vi "load modules.vi"() -> ()   [LabVIEW 2012]
uses:
  GFG/GFGstringGet.vi
  GFG/GFG library.lvlib
panel:
  out "Array":T1(array[cluster])
  out "error out":errorcluster
  in  "error in (no error)":errorcluster
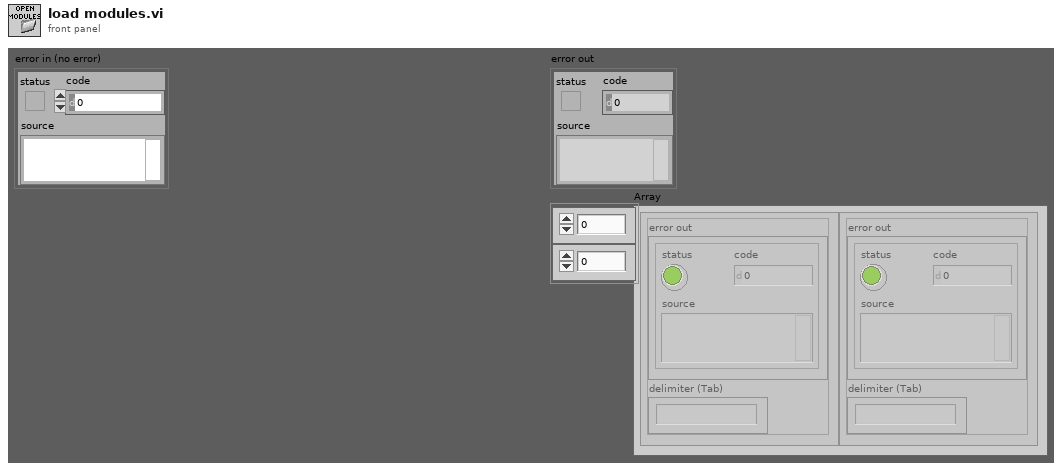
[diagram p1: front panel]
types:
  T1 = cluster{"error out":errorcluster, "delimiter (Tab)":string}[][]
  T2 = enum32{"Invalid", "Standard", "Closed", "Hidden", "Minimized", "Maximized"}
  T3 = cluster{"error out":errorcluster, "delimiter (Tab)":string}
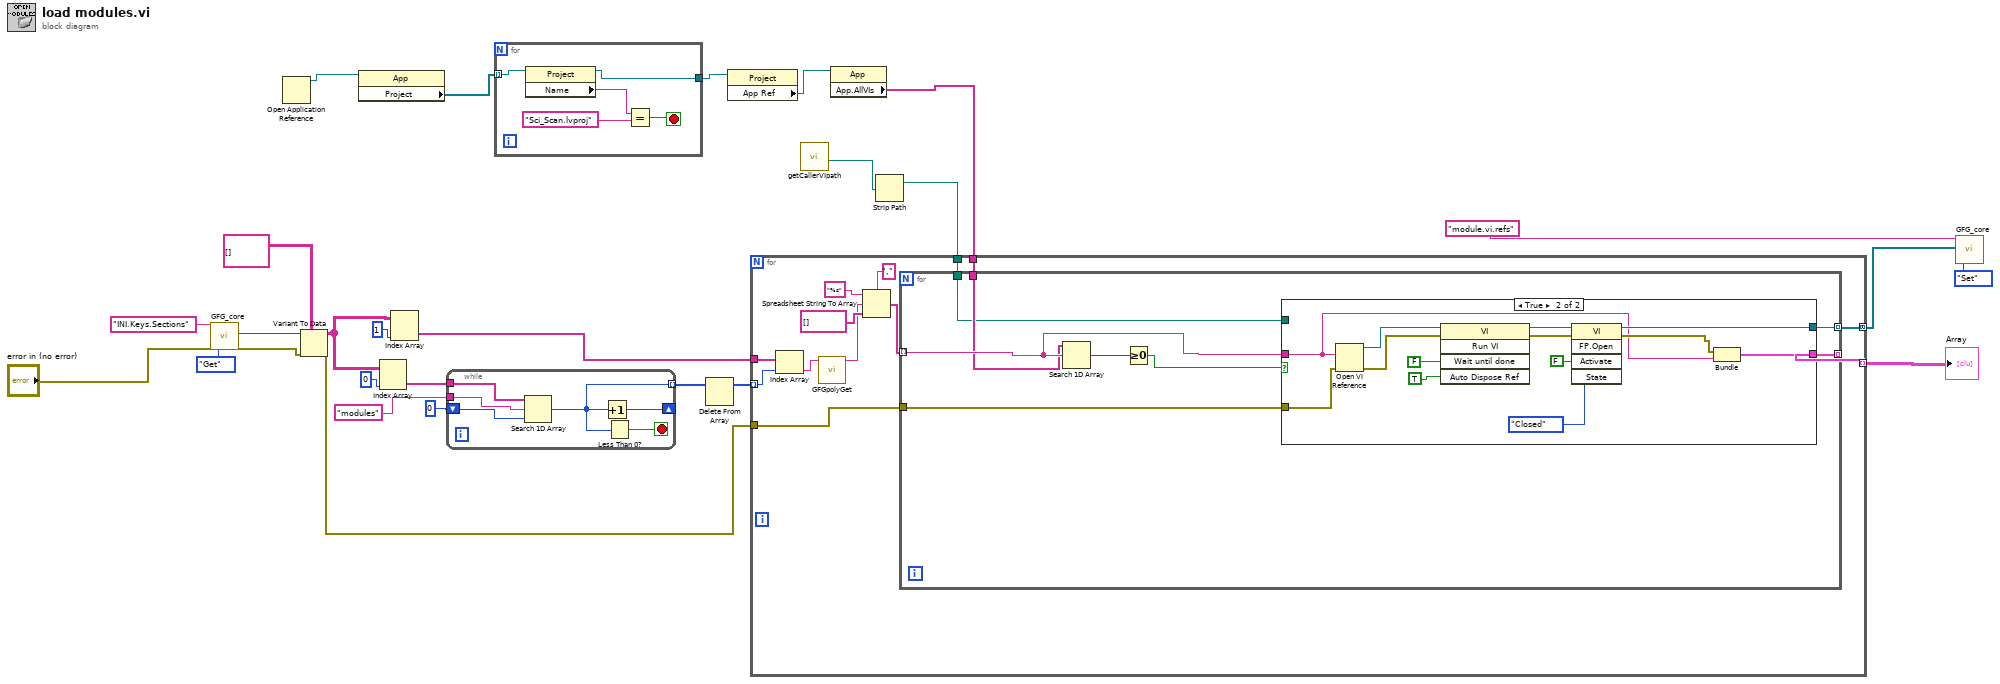
[diagram p0: block diagram]
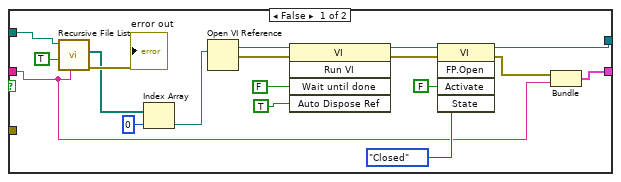
[diagram p2: hidden frame]
diagram:
  n1 = call "GFG_core.vi"("Variable Name in"="INI.Keys.Sections", "error in (no error)"="error in (no error)", "Action"=enum16{"Init", "Set", "Get"}."Get") -> ("Variant Out"=w25:variant, "error out"=w13:errorcluster)  [unwired: 10 in, 5 out]
  n2 = Open Application Reference() -> (3:w2:refnum<vi>)  [unwired: 4 in, 1 out]
  n3 = Variant To Data(error in=w13, type=string[][] [], Variant=w25) -> (data=w21:string[][], error out=w12:errorcluster)
  n4 = property class="App"(reference=w2) -> ("Project"=w3:refnum<vi>[])  [unwired: 1 in, 2 out]
  n5 = Index Array(array=w21, index (col)=0 ("index (row)")) -> (element=w23:string[])  [unwired: 1 in]
  n6 = Index Array(array=w21, index (col)=1 ("index (row)")) -> (element=w20:string[])  [unwired: 1 in]
  n7 = while {
    tunnel: w23 -> [w33]
    shift-right: [w30] -> _
    shift-left: 0 ("index of element") -> [w32]
    tunnel: [w29] -> w16 mode=indexing
    tunnel: "modules" ("element") -> [w28]
    stop <- w31 stop-if-true
    n8 = Search 1D Array(1D array=w33, element=w28, start index (0)=w32) -> (index of element=w29:i32)
    n9 = Increment(x=w29) -> (x+1=w30:i32)
    n10 = Less Than 0?(x=w29) -> (x < 0?=w31:bool)
  }
  n11 = for {
    tunnel: w3 -> [w38] mode=indexing
    tunnel: [w35] -> w4
    stop <- w34 stop-if-true
    n12 = property class="Project"(reference=w38) -> (reference out=w35:refnum<vi>, "Name"=w36:string)  [unwired: 1 in, 1 out]
    n13 = Equal?(x=w36, y="Sci_Scan.lvproj" ("Name")) -> (x = y?=w34:bool)
  }
  n14 = Delete From Array(array=w16) -> (array with subset deleted=w15:i32[])  [unwired: 2 in, 1 out]
  n15 = property class="Project"(reference=w4) -> ("App Ref"=w5:refnum<vi>)  [unwired: 1 in, 2 out]
  n16 = call "getCallerVIpath.vi"() -> ("calling VI's  parent path"=w7:path)  [unwired: 10 in, 1 out]
  n17 = property class="App"(reference=w5) -> ("App.AllVIs"=w1:string[])  [unwired: 1 in, 2 out]
  n18 = Strip Path(path=w7) -> (stripped path=w6:path)  [unwired: 1 out]
  n19 = for {
    tunnel: w20 -> [w51]
    tunnel: w15 -> [w50] mode=indexing
    tunnel: w12 -> [w49]
    tunnel: [w42] -> w10 mode=concatenating
    tunnel: w6 -> [w41]
    tunnel: [w40] -> w8 mode=indexing
    tunnel: w1 -> [w39]
    n20 = Index Array(array=w51, index=w50) -> (element=w44:string)
    n21 = call-poly "GFGpolyGet.vi"("Variable Name in"=w44) -> ("String"=w43:string)  [unwired: 10 in]
    n22 = Spreadsheet String To Array(delimiter (Tab)=",", format string="%s" ("Variable Name in"), spreadsheet string=w43, array type (2D Dbl)=string[] [] ("Array")) -> (array=w45:string[])
    n23 = for {
      tunnel: w49 -> [w54]
      tunnel: w45 -> [w57] mode=indexing
      tunnel: [w59] -> w42 mode=indexing
      tunnel: w41 -> [w53]
      tunnel: [w58] -> w40 mode=indexing
      tunnel: w39 -> [w56]
      n24 = Search 1D Array(1D array=w56, element=w57) -> (index of element=w52:i32)  [unwired: 1 in]
      n25 = Greater Or Equal To 0?(x=w52) -> (x >= 0?=w55:bool)
      n26 = case shown="True" w55 {
        tunnel: w54 -> [_ w86]
        tunnel: [w61 w85] -> w59
        tunnel: [w60 w84] -> w58
        tunnel: w57 -> [w62 w78]
        tunnel: w53 -> [w73 _]
        frame False {
          n27 = call <vilib>:"Recursive File List.vi"("pattern"=w62, "Continue Recursing on Error? (F)"=TRUE, "Folder Path"=w73) -> ("error out"=→"error out":errorcluster, "All Files in Dir"=w75:path[])  [unwired: 4 in, 3 out]
          n28 = Index Array(array=w75, index=0) -> (element=w63:path)
          n29 = Open VI Reference(vi path=w63) -> (vi reference=w67:refnum<vi>, error out=w72:errorcluster)  [unwired: 5 in]
          n30 = invoke class="VI" method="Run VI"(reference=w67, error in=w72, "Wait until done"=FALSE, "Auto Dispose Ref"=TRUE ("Auto Dispose Reference")) -> (reference out=w65:refnum<vi>, error out=w70:errorcluster)  [unwired: 1 in, 3 out]
          n31 = invoke class="VI" method="FP.Open"(reference=w65, error in=w70, "Activate"=FALSE ("Activate?"), "State"=T2."Closed") -> (reference out=w61:refnum<vi>, error out=w71:errorcluster)  [unwired: 1 in, 3 out]
          n32 = Bundle("error out"=w71, "delimiter (Tab)"=w62) -> (w60:T3)  [unwired: 1 in]
        }
        frame True {
          n33 = Open VI Reference(vi path=w78, error in (no error)=w86) -> (vi reference=w87:refnum<vi>, error out=w79:errorcluster)  [unwired: 4 in]
          n34 = invoke class="VI" method="Run VI"(reference=w87, error in=w79, "Wait until done"=FALSE, "Auto Dispose Ref"=TRUE ("Auto Dispose Reference")) -> (reference out=w89:refnum<vi>, error out=w81:errorcluster)  [unwired: 1 in, 3 out]
          n35 = invoke class="VI" method="FP.Open"(reference=w89, error in=w81, "Activate"=FALSE ("Activate?"), "State"=T2."Closed") -> (reference out=w85:refnum<vi>, error out=w80:errorcluster)  [unwired: 1 in, 3 out]
          n36 = Bundle("error out"=w80, "delimiter (Tab)"=w78) -> (w84:T3)  [unwired: 1 in]
        }
      }
    }
  }
  "Array" <- w8
  n37 = call "GFG_core.vi"("Variable Name in"="module.vi.refs", "Variant in"=w10, "Action"=enum16{"Init", "Set", "Get"}."Set") -> ()  [unwired: 10 in, 7 out]
